vi "15T_Check_Queue.vi"(7 "error in (no error)":errorcluster caption="Fehler (Eingang, kein Fehler)", 10 "queue":refnum<queue>) -> (0 "error out":errorcluster caption="Fehler (Ausgang)", 1 "15T-Control":T1={"Setpoint (T)"=3.4572, "Rate (T/min)"=0.0, "Go to zero"=FALSE, "Go to Hold"=FALSE, "Go to Set"=FALSE, "Clamp"=FALSE, "Switch Heater"=FALSE} {"Rate (T/min)" format="%6_5f"; "Setpoint (T)" format="%6_5f"}, 3 "New Entries?":bool)   [LabVIEW 2018]
uses:
  Berta/15T-Control.ctl
panel:
  out "Numeric":i32
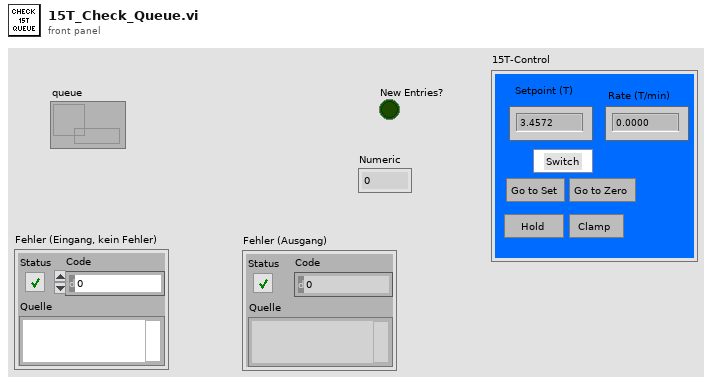
[diagram p1: front panel]
types:
  T1 = typedef "15T-Control.ctl" = cluster{"Setpoint (T)":dbl, "Rate (T/min)":dbl, "Go to zero":bool, "Go to Hold":bool, "Go to Set":bool, "Clamp":bool, "Switch Heater":bool}
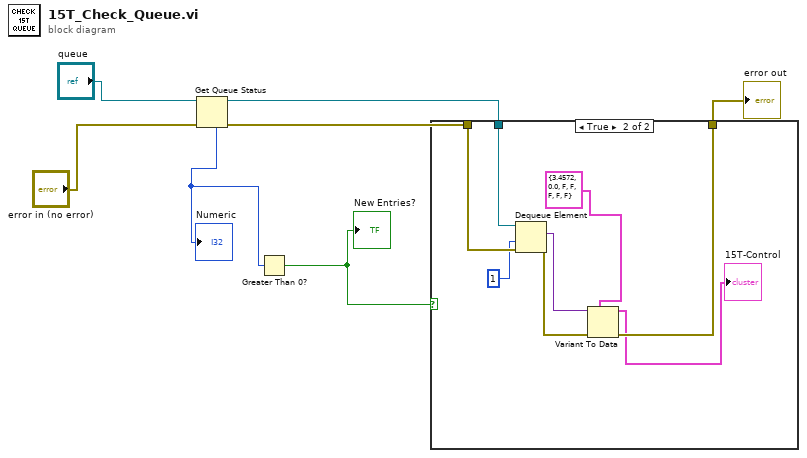
[diagram p0: block diagram]
diagram:
  n1 = Get Queue Status(queue="queue", error in (no error)="error in (no error)") -> (queue out=w5:refnum<queue>, error out=w4:errorcluster, # elements in queue=w3:i32)  [unwired: 1 in, 5 out]
  "Numeric" <- w3
  n2 = Greater Than 0?(x=w3) -> (x > 0?=w2:bool)
  "New Entries?" <- w2
  n3 = case shown="True" w2 {
    tunnel: w5 -> [_ w16]
    tunnel: w4 -> [w8 w15]
    tunnel: [w8 w12] -> w1
    frame False {
    }
    frame True {
      n4 = Dequeue Element(queue=w16, timeout in ms (-1)=1, error in (no error)=w15) -> (element=w13:variant, error out=w11:errorcluster)  [unwired: 2 out]
      n5 = Variant To Data(error in=w11, type=T1 {"Setpoint (T)"=3.4572, "Rate (T/min)"=0.0, "Go to zero"=FALSE, "Go to Hold"=FALSE, "Go to Set"=FALSE, "Clamp"=FALSE, "Switch Heater"=FALSE} ("15T-Control"), Variant=w13) -> (data=→"15T-Control":T1, error out=w12:errorcluster)
    }
  }
  "error out" <- w1
